vi "AMZ_S3_SHA-256.vi"(11 "Message":string) -> (3 "Hash Value":string)   [LabVIEW 2015, in "LV Interface for Amazon S3.lvlib"]
doc: "Calculates a hash for the given <b>Message</b>.\n\n(c) Ton Plomp, 2011\nTHIS SOFTWARE IS PROVIDED AS IS, AND ANY WARRANTY IS REJECTED"
uses:
  LV Interface for Amazon S3.lvlib
  <vilib>/LVH/i3 External Encryption/i3-external-encryption.lvlib
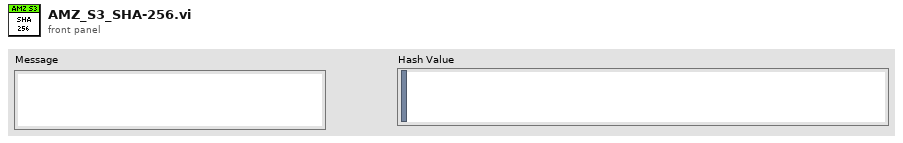
[diagram p1: front panel]
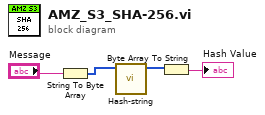
[diagram p0: block diagram]
diagram:
  n1 = String To Byte Array(string="Message") -> (unsigned byte array=w4:u8[])
  n2 = call <vilib>:"Hash-string.vi"("Message"=w4) -> ("Hash"=w2:u8[])  [unwired: 8 in, 2 out]
  n3 = Byte Array To String(unsigned byte array=w2) -> (string=→"Hash Value":string)
